vi "get available properties.vi"(8 "error in":errorcluster, 9 "propertynode_id":string) -> (0 "error out":errorcluster, 3 "All Supported Properties":T1)   [LabVIEW 2020]
doc: "Returns the available property IDs for a Property Node -- this does not work on Invoke Nodes (use set_invoke_node for those instead). Use this before set_property to find the correct property ID. Make sure a concrete-class reference (VI, Control, Application, etc.) is already wired into the property node's input, since the available properties depend on that class."
uses:
  <vilib>/_script/All Supported PropertiesOrMethods TypeDefs/ASPM_ArrayOfUniqueIDStringDatanameShortnameLongname.ctl
  <vilib>/_script/All Supported PropertiesOrMethods TypeDefs/ASPM_UniqueIDStringDatanameShortnameLongname.ctl
  G-AI Core/G-AI Core.lvlib
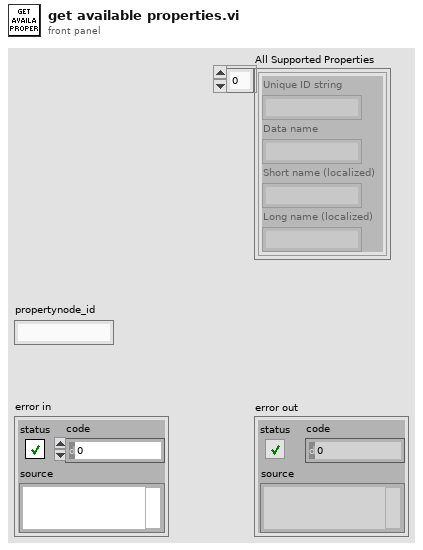
[diagram p1: front panel]
types:
  T1 = typedef "ASPM_ArrayOfUniqueIDStringDatanameShortnameLongname.ctl" = T2[]
  T2 = typedef "ASPM_UniqueIDStringDatanameShortnameLongname.ctl" = cluster{"Unique ID string":string, "Data name":string, "Short name (localized)":string, "Long name (localized)":string}
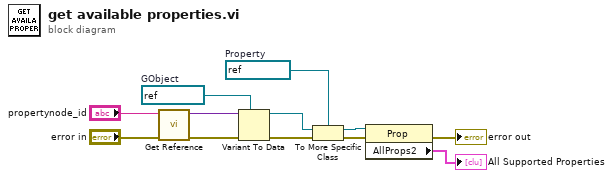
[diagram p0: block diagram]
diagram:
  w7 = refnum<vi> refnum  # Property
  w8 = refnum<vi> refnum  # GObject
  n1 = call "Get Reference.vi"("error in"="error in", "id"="propertynode_id") -> ("error out"=w11:errorcluster, "reference"=w10:variant)  [unwired: 8 in]
  n2 = Variant To Data(error in=w11, type=w8, Variant=w10) -> (data=w6:refnum<vi>, error out=w9:errorcluster)
  n3 = To More Specific Class(target class=w7, reference=w6, error in=w9) -> (specific class reference=w3:refnum<vi>, error out=w5:errorcluster)
  n4 = property class="Prop"(reference=w3, error in=w5) -> (error out=→"error out":errorcluster, "AllProps2"=→"All Supported Properties":T1)  [unwired: 1 out]
